vi "Insert Stop Loop.vi"(6 "Insertion Index":i32=-1, 7 "Parent ID":string, 8 "error in (no error)":errorcluster, 9 "Unique ID":string, 10 "Name":string, 11 "Test Executive in":refnum<class "Test Executive.lvclass">) -> (0 "error out":errorcluster, 1 "Replaced?":bool, 3 "Test Executive out":refnum<class "Test Executive.lvclass">, 5 "Unique ID out":string)   [LabVIEW 2019, in "Test Executive.lvlib" / "Test Executive.lvclass"]
uses:
  <vilib>/gpm_packages/@cs/test-executive/Source/Test Executive/TestExecutive/Test Executive.lvclass
  <vilib>/gpm_packages/@cs/test-executive/Source/Test Executive/Stop Loop/Stop Loop.lvclass
  <vilib>/gpm_packages/@cs/test-executive/Source/Test Executive/TestExecutive/Test Executive.lvclass/Test Executive.ctl
  <vilib>/gpm_packages/@cs/linked-list/Source/Linked List/Linked List Ref/Linked List Ref.lvclass
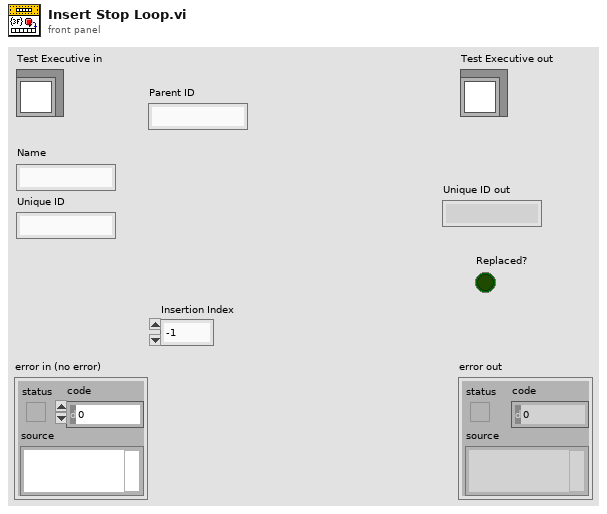
[diagram p1: front panel]
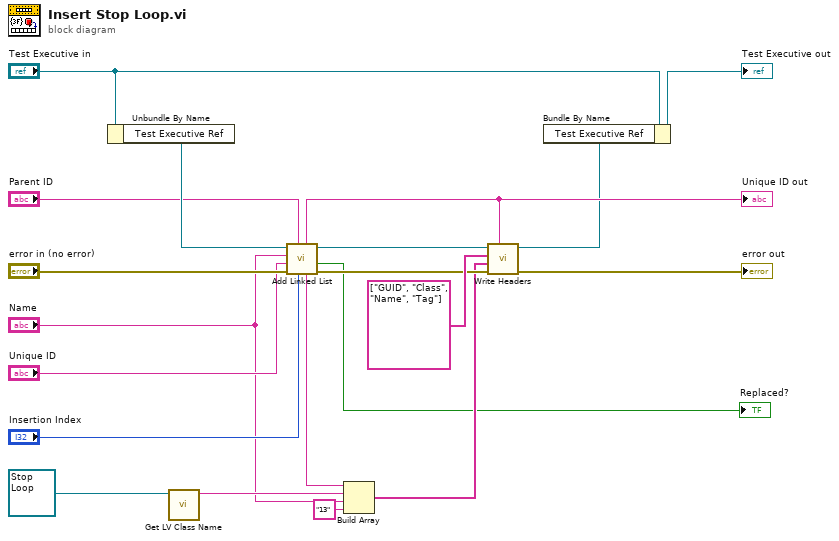
[diagram p0: block diagram]
diagram:
  n1 = Unbundle By Name("Test Executive in") -> ("Test Executive Ref"=w14:refnum<data-value>)
  n2 = call <vilib>:"Get LV Class Name.vi"("object"=refnum<class "Stop Loop.lvclass"> refnum ("Test Executive.lvlib:Stop Loop.lvclass")) -> ("class name"=w11:string)  [unwired: 9 in, 1 out]
  n3 = call <vilib>:"Add Linked List.vi"("Insertion Index"="Insertion Index", "Parent ID"="Parent ID", "error in (no error)"="error in (no error)", "Linked List ID"="Unique ID", "Name"="Name", "Linked List Ref"=w14) -> ("error out"=w16:errorcluster, "Replaced?"=→"Replaced?":bool, "Linked List Ref out"=w13:refnum<data-value>, "Linked List ID out"=w4:string)  [unwired: 2 in]
  "Unique ID out" <- w4
  n4 = Build Array(w4, w11, "Name", "13" ("element")) -> (w15:string[])
  n5 = call <vilib>:"Write Headers.vi"("Linked List ID"=w4, "error in (no error)"=w16, "Header Values"=w15, "Header Names"=string[] ["GUID", "Class", "Name", "Tag"], "Linked List Ref"=w13) -> ("error out"=→"error out":errorcluster, "Linked List Ref out"=w3:refnum<data-value>)  [unwired: 5 in]
  n6 = Bundle By Name(cluster="Test Executive in", "Test Executive Ref"=w3) -> (→"Test Executive out":refnum<class "Test Executive.lvclass">)
